vi "Append File to Report.vi"(0 "report in":refnum<class "NI_Standard Report.lvclass">, 1 "MS Office parameters":T1, 7 "file path":path, 9 "is spreadsheet file? (Excel)":bool, 11 "error in (no error)":errorcluster) -> (4 "report out":refnum<class "NI_Standard Report.lvclass">, 8 "start out (Word)":i32, 10 "end out (Word)":i32, 15 "error out":errorcluster)   [LabVIEW 2015, in "NI_Standard Report.lvclass"]
doc: "Appends the text from a text file into the current report."
uses:
  <vilib>/Utility/NIReport.llb/Standard Report/NI_Standard Report.lvclass
  <vilib>/Utility/NIReport.llb/Standard Report/NI_Standard Report.lvclass/NI_Standard Report.ctl
  <vilib>/Utility/NIReport.llb/NI_ReportGenerationCore.lvlib
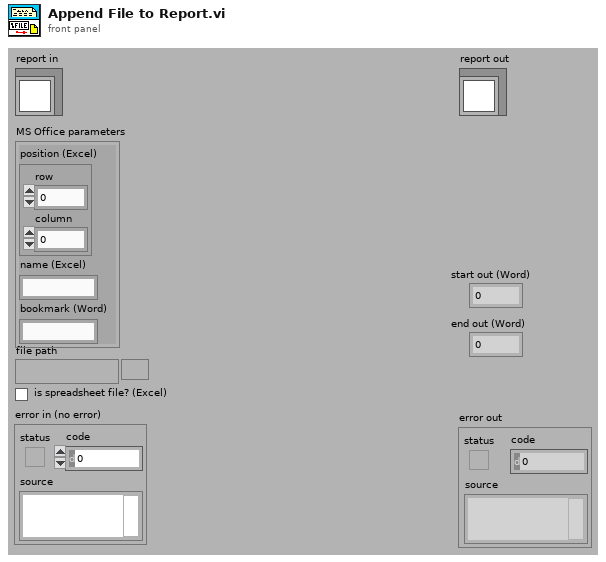
[diagram p1: front panel]
types:
  T1 = cluster{"position (Excel)":cluster{"row":i32, "column":i32}, "name (Excel)":string, "bookmark (Word)":string}
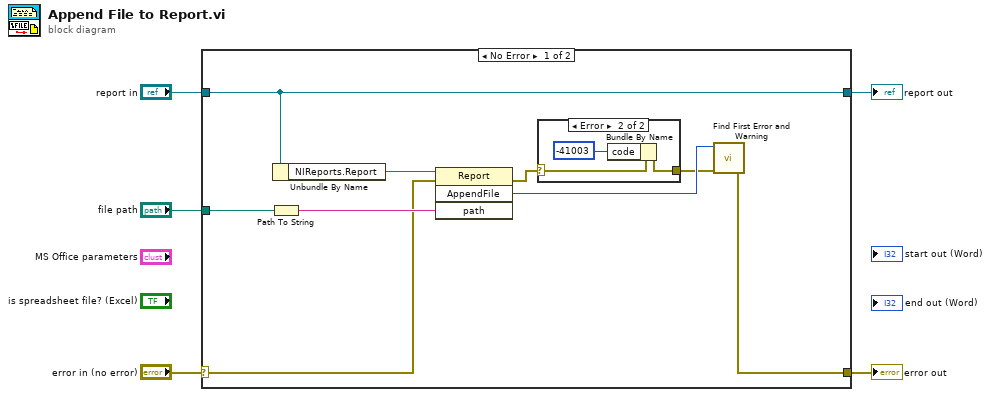
[diagram p0: block diagram]
diagram:
  n1 = case shown="No Error" "error in (no error)" {
    selector: "error in (no error)" -> [w7 w20]
    tunnel: [w6 w20] -> w4
    tunnel: [w9 w19] -> w2
    tunnel: "report in" -> [w9 w19]
    tunnel: "file path" -> [w8 _]
    frame No Error {
      n2 = Path To String(path=w8) -> (string=w11:string)
      n3 = Unbundle By Name(w9) -> ("NIReports.Report"=w12:refnum<k7>)
      n4 = invoke class="Report" method="AppendFile"(reference=w12, error in=w7, "path"=w11) -> (error out=w10:errorcluster, "AppendFile"=w14:i32)  [unwired: 1 in, 2 out]
      n5 = case shown="Error" w10 {
        selector: w10 -> [w15 w16]
        tunnel: [w15 w17] -> w13
        frame No Error {
        }
        frame Error {
          n6 = Bundle By Name(cluster=w16, "code"=-41003) -> (w17:errorcluster)
        }
      }
      n7 = call <vilib>:"Find First Error and Warning.vi"("error in (no error)"=w13, "error code"=w14) -> ("error out"=w6:errorcluster)  [unwired: 1 in, 4 out]
    }
    frame Error {
    }
  }
  "error out" <- w4
  "report out" <- w2
